vi "Cleanup Default Value Template.vi"(8 "error in":errorcluster, 10 "temporary template path":path, 11 "gRPCid in":T1) -> (0 "error out":errorcluster)   [LabVIEW 2021, in "MeasurementClient Editor.lvlib"]
uses:
  MeasurementClient Editor.lvlib
  <vilib>/gRPC/LabVIEW gRPC Library/Shared/grpcId.ctl
  <vilib>/gRPC/Generated APIs/ni/measurementlink/measurement/v2/Measurement Service Client V2/Measurement Service Client V2.lvlib
  <vilib>/gRPC/LabVIEW gRPC Library/grpc-lvsupport-release.lvlib
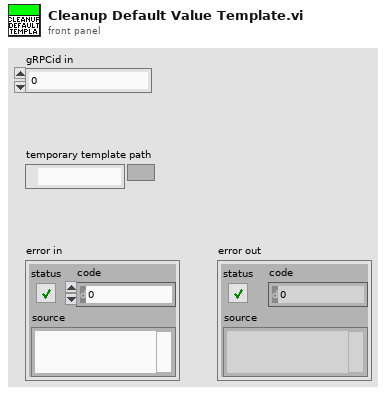
[diagram p1: front panel]
types:
  T1 = typedef "grpc-lvsupport-release.lvlib/grpcId.ctl" = u64
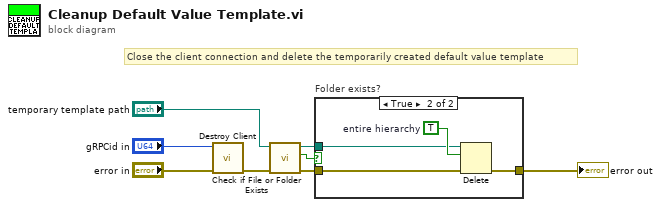
[diagram p0: block diagram]
diagram:
  # "Close the client connection and delete the temporarily created default value template"
  n1 = call <vilib>:"Destroy Client.vi"("error in"="error in", "gRPC ID"="gRPCid in") -> ("error out"=w4:errorcluster)  [unwired: 9 in]
  n2 = call <vilib>:"Check if File or Folder Exists.vi"("error in (no error)"=w4, "path"="temporary template path") -> ("error out"=w3:errorcluster, "file or folder exists?"=w2:bool, "dup path"=w1:path)  [unwired: 7 in]
  n3 = case "Folder exists?" shown="True" w2 {
    tunnel: [w9 w10] -> w7
    tunnel: w3 -> [w9 w11]
    tunnel: w1 -> [_ w12]
    frame False {
    }
    frame True {
      w13 = TRUE  # entire hierarchy
      n4 = Delete(path (use dialog)=w12, entire hierarchy (F)=w13, error in=w11) -> (error out=w10:errorcluster)  [unwired: 2 in, 2 out]
    }
  }
  "error out" <- w7
